vi "SVT Phase Linearity.vi"   [LabVIEW 2017, in "SoundVib_Distortion.lvlib"]
doc: "Computes the multitone phase of each tone in a multitone signal, the average group delay, and the max deviation of the phase from a straight line. Use a square wave or construct the input signal with component tones evenly spaced in frequency and with zero relative phase between the component tones."
uses:
  <vilib>/addons/Sound and Vibration/svt_Distortion/SoundVib_Distortion.lvlib
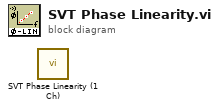
[diagram p0: block diagram]
diagram:
  n1 = call <vilib>:"SVT Phase Linearity (1 Ch).vi"() -> ()  [unwired: 11 in, 9 out]
